vi "Image rotate and merge Main.vi"() -> ()   [LabVIEW 2016]
uses:
  <vilib>/vision/NI_Vision_Development_Module.lvlib
panel:
  out "最終角度":i32
  out "圖片數":i32
  in  "預設旋轉的步進角度":sgl=5.0
  out "提取範圍":T1(plugin-control)
  in  "預設 ROI":T2={"Rectangle"=[23, 116, 62, 596], "Contours"=[{"Type"=0, "ROI Type"=3, "Points"=[23, 116, 62, 596]}]}
  out "步進角度":sgl=3.8
  out "圖像中心位置":i32[](array[numeric])=[337, 356]
  out "圖像旋轉":T1(plugin-control)
  out "旋轉角度":sgl=22.8
  out "圖像合併":T1(plugin-control)
  in  "wait":u32=1000
  out "原始圖":T1(plugin-control)
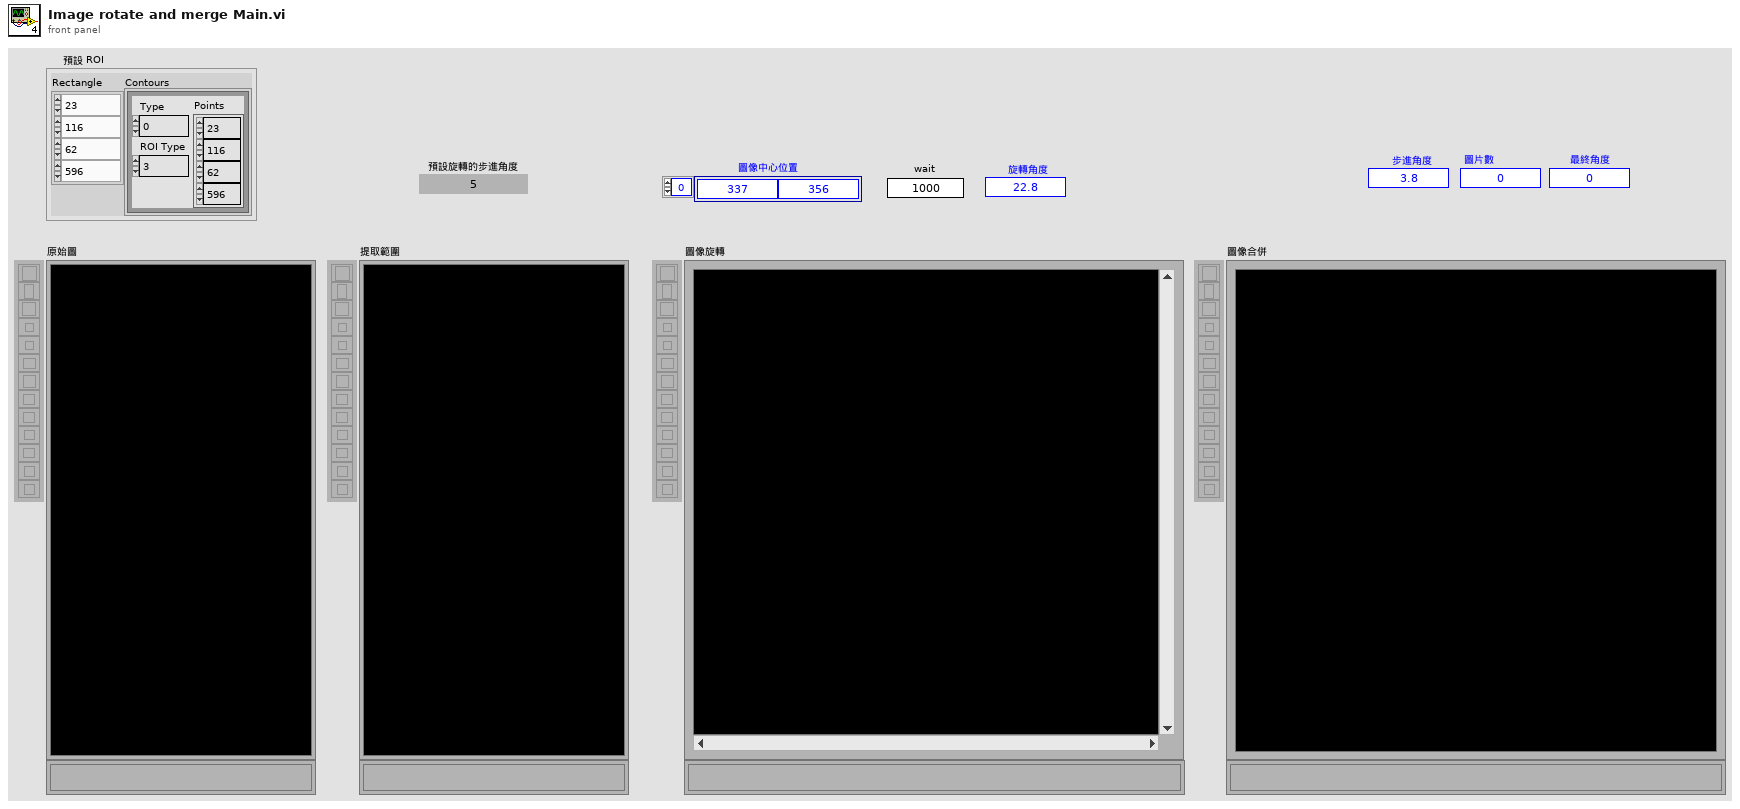
[diagram p1: front panel]
types:
  T1 = typedef "IMAQ Image.ctl" = refnum<image>
  T2 = cluster{"Rectangle":i32[], "Contours":cluster{"Type":u32, "ROI Type":u32, "Points":i32[]}[]}
  T3 = enum32{"Invalid", "Standard", "Closed", "Hidden", "Minimized", "Maximized"}
  T4 = cluster{"This VI":refnum<vi>, "path":path, "提取扇形矩形輪廓":i32[], "Roi 參數":cluster{"Left":i32, "Top":i32, "Right":i32, "Bottom":i32, "旋轉角度":sgl}, "中心點":cluster{"X":i32, "Y":i32}, "預設圖框":u8[][], "步進角度":sgl}
  T5 = cluster{"Global Rectangle":i32[], "Contours":cluster{"Contour Type":u32, "ROI Type":u32, "Points":i32[]}[]}
  T6 = typedef "IMAQ Rectangle" = cluster{"Left":i32, "Top":i32, "Right":i32, "Bottom":i32, "Rotation":dbl}
  T7 = typedef "Image Type" = u32
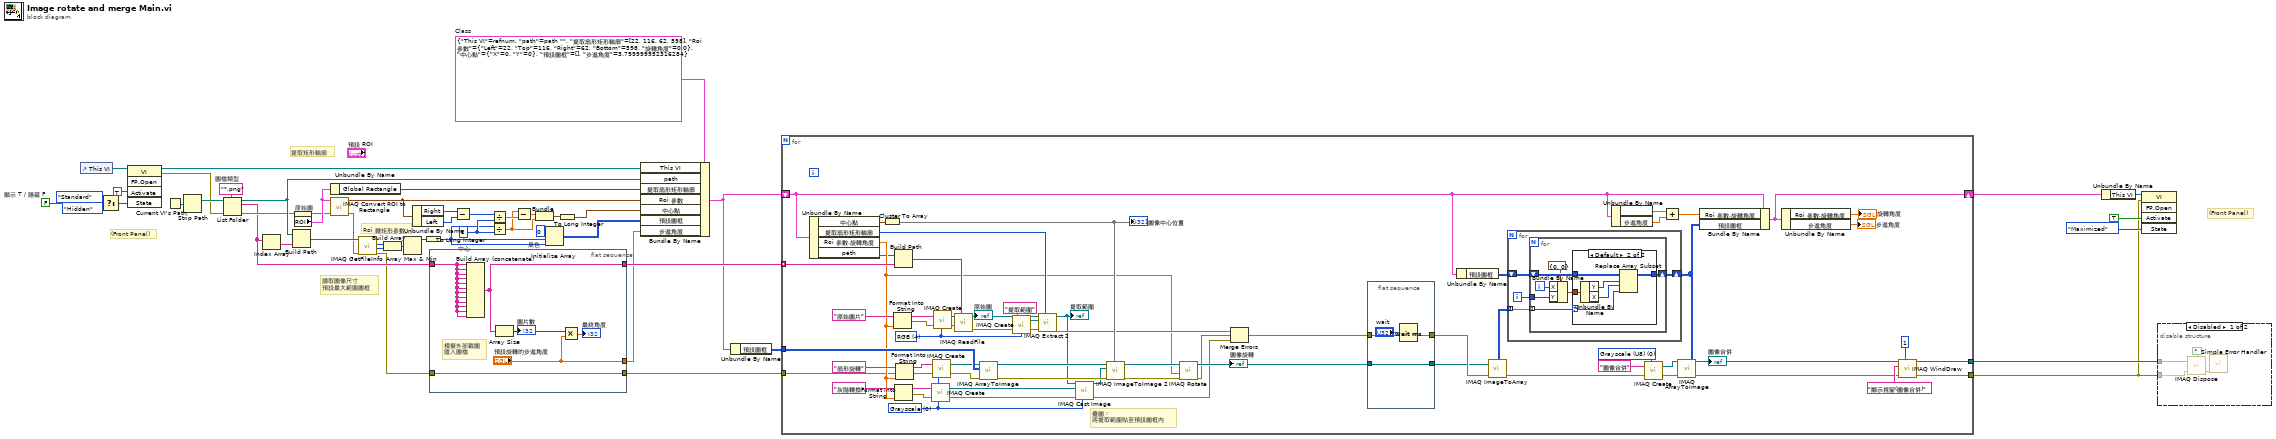
[diagram p0: block diagram]
diagram:
  w8 = FALSE  # 顯示 T / 隱藏 F
  w36 = 2  # 中心
  w42 = u8 0  # 黑色
  w28 = T4 {"This VI"=refnum, "path"=path "", "提取扇形矩形輪廓"=[22, 116, 62, 598], "Roi 參數"={"Left"=22, "Top"=116, "Right"=62, "Bottom"=598, "旋轉角度"=0.0}, "中心點"={"X"=0, "Y"=0}, "預設圖框"=[], "步進角度"=3.8}  # Class
  w48 = "*.png"  # 圖檔類型
  # "(Front Panel)"
  # "Roi 轉矩形參數"
  # "讀取圖像尺寸\n預設最大範圍圖框"
  # "(Front Panel)"
  # "提取矩形輪廓"
  n1 = control-ref of="This VI"() -> (w34:refnum<vi>)
  n2 = Select(t=T3."Standard" ("State"), s=w8, f=T3."Hidden" ("State")) -> (s? t:f=w5:T3)
  n3 = invoke class="VI" method="FP.Open"(reference=w34, "Activate"=TRUE ("Activate?"), "State"=w5) -> (reference out=w27:refnum<vi>, error out=w25:errorcluster)  [unwired: 2 in, 3 out]
  n4 = Current VI's Path() -> (path=w50:path)
  n5 = Strip Path(path=w50) -> (stripped path=w49:path)  [unwired: 1 out]
  n6 = List Folder(path=w49, pattern=w48, error in=w25) -> (path out=w26:path, filenames=w15:string[], error out=w23:errorcluster)  [unwired: 1 in, 1 out]
  n7 = Index Array(array=w15) -> (element=w47:string)  [unwired: 1 in]
  n8 = Build Path(base path=w26, name or relative path=w47) -> (appended path=w46:path)
  n9 = property on="原始圖" class="ImageControl"(error in=w23) -> (error out=w22:errorcluster, "ROI"=w24:T5)  [unwired: 1 in, 1 out]
  n10 = Unbundle By Name(w24) -> ("Global Rectangle"=w21:i32[])
  n11 = call "IMAQ Convert ROI to Rectangle"("error in (no error)"=w22, "ROI Descriptor"=w24) -> ("error out"=w4:errorcluster, "Rectangle"=w20:T6)  [unwired: 7 in]
  n12 = call "IMAQ GetFileInfo"("error in (no error)"=w4, "File Path"=w46) -> ("error out"=w3:errorcluster, "Y Resolution"=w43:i32, "X Resolution"=w45:i32)  [unwired: 3 in, 4 out]
  n13 = Build Array(w45, w43) -> (w44:i32[])
  n14 = Array Max & Min(array=w44) -> (max value=w41:i32)  [unwired: 3 out]
  n15 = Unbundle By Name(w20) -> ("Right"=w40:i32, "Left"=w39:i32)
  n16 = To Long Integer(number=w41) -> (32bit integer=w35:i32)
  n17 = flat-sequence {
    tunnel: w15 -> [w55]
    tunnel: [w53] -> w14
    tunnel: [w56] -> w13
    tunnel: w3 -> [w56]
    tunnel: ["預設旋轉的步進角度"] -> w9
    frame #0 {
      # "模擬外部截圖\n匯入圖檔"
      n18 = Build Array (concatenate)(w55, w55, w55, w55, w55, w55, w55, w55, w55, w55, w55, w55) -> (w53:string[])
      n19 = Array Size(array=w53) -> (size(s)=w54:i32)
      "圖片數" <- w54
      n20 = Multiply(x=w54, y="預設旋轉的步進角度") -> (x*y=→"最終角度":sgl)
    }
  }
  n21 = Subtract(x=w40, y=w39) -> (x-y=w38:i32)
  n22 = Divide(x=w38, y=w36) -> (x/y=w37:dbl)
  n23 = Divide(x=w35, y=w36) -> (x/y=w18:dbl)
  n24 = Subtract(x=w18, y=w37) -> (x-y=w19:dbl)
  n25 = Bundle(w19, w18) -> (w17:cluster{dbl, dbl})  [unwired: 1 in]
  n26 = Initialize Array(w42, w35, w35) -> (w11:u8[][])
  n27 = To Long Integer(number=w17) -> (32bit integer=w16:cluster{i32, i32})
  n28 = Bundle By Name(cluster=w28, "This VI"=w27, "path"=w26, "提取扇形矩形輪廓"=w21, "Roi 參數"=w20, "中心點"=w16, "預設圖框"=w11, "步進角度"=w9) -> (w12:T4)
  n29 = Unbundle By Name(w12) -> ("預設圖框"=w10:u8[][])
  n30 = for {
    tunnel: w14 -> [w115] mode=indexing
    tunnel: [w58] -> w1
    shift-right: [w70] -> w30
    shift-left: w12 -> [w93]
    tunnel: w10 -> [w92]
    tunnel: [w59] -> w2
    tunnel: w13 -> [w81]
    w110 = T7 0 items=["Grayscale (U8)", "Grayscale (I16)", "Grayscale (SGL)", "Complex (CSG)", "RGB (U32)", "HSL (U32)", "RGB (U64)", "Grayscale (U16)"] ("Image Type")
    w97 = T7 0 items=["Grayscale", "Grayscale (I16)", "Grayscale (SGL)", "Complex (CSG)", "RGB (U32)", "HSL (U32)", "RGB (U64)", "Grayscale (U16)"] ("Image Type")
    w71 = T7 4 items=["Grayscale (U8)", "Grayscale (I16)", "Grayscale (SGL)", "Complex (CSG)", "RGB", "HSL (U32)", "RGB (U64)", "Grayscale (U16)"] ("Image Type")
    # "疊圖 :\n將提取範圍貼至預設圖框內"
    n31 = Unbundle By Name(w93) -> ("中心點"=w85:cluster{"X":i32, "Y":i32}, "提取扇形矩形輪廓"=w84:i32[], "Roi 參數.旋轉角度"=w83:sgl, "path"=w82:path)
    n32 = Cluster To Array(cluster=w85) -> (array=w87:i32[])
    "圖像中心位置" <- w87
    n33 = Format Into String(initial string="原始圖片" ("Image Name"), w83) -> (resulting string=w120:string, error out=w119:errorcluster)  [unwired: 2 in]
    n34 = Format Into String(initial string="灰階轉換" ("Image Name"), w83) -> (resulting string=w117:string, error out=w116:errorcluster)  [unwired: 2 in]
    n35 = Build Path(base path=w82, name or relative path=w115) -> (appended path=w114:path)
    n36 = Format Into String(initial string="扇形旋轉" ("Image Name"), error in=w81, w83) -> (resulting string=w101:string, error out=w100:errorcluster)  [unwired: 1 in]
    n37 = call "IMAQ Create"("Image Name"=w117, "Image Type"=w97, "error in (no error)"=w116) -> ("New Image"=w111:T1, "error out"=w89:errorcluster)  [unwired: 1 in, 1 out]
    n38 = call "IMAQ Create"("Image Name"=w101, "Image Type"=w97, "error in (no error)"=w100) -> ("New Image"=w74:T1, "error out"=w103:errorcluster)  [unwired: 1 in, 1 out]
    n39 = call "IMAQ Create"("Image Name"=w120, "Image Type"=w71, "error in (no error)"=w119) -> ("New Image"=w113:T1, "error out"=w112:errorcluster)  [unwired: 2 in]
    n40 = call "IMAQ ReadFile"("File Path"=w114, "error in (no error)"=w112, "Image"=w113) -> ("error out"=w67:errorcluster, "Image Out"=w75:T1)  [unwired: 4 in, 3 out]
    "原始圖" <- w75
    n41 = call "IMAQ ArrayToImage"("error in (no error)"=w103, "Image Pixels (U8)"=w92, "Image"=w74) -> ("error out"=w98:errorcluster, "Image Out"=w99:T1)  [unwired: 7 in]
    n42 = call "IMAQ Create"("Image Name"="提取範圍", "Image Type"=w71, "error in (no error)"=w67) -> ("New Image"=w72:T1, "error out"=w66:errorcluster)  [unwired: 2 in]
    n43 = call "IMAQ Extract 2"("Optional Rectangle"=w84, "error in (no error)"=w66, "Image Dst"=w72, "Image Src"=w75) -> ("error out"=w86:errorcluster, "Image Dst Out"=w65:T1)  [unwired: 6 in]
    "提取範圍" <- w65
    n44 = call "IMAQ Cast Image"("Image Type"=w97, "error in (no error)"=w89, "Image Dst"=w111, "Image Src"=w65) -> ("error out"=w63:errorcluster, "Image Dst Out"=w73:T1)  [unwired: 6 in]
    n45 = call "IMAQ ImageToImage 2"("Offset Left/Top"=w87, "error in (no error)"=w98, "Image Src (Small)"=w73, "Image Src (Large)"=w99) -> ("error out"=w104:errorcluster, "Image Dst Out"=w105:T1)  [unwired: 6 in]
    n46 = call "IMAQ Rotate"("error in (no error)"=w104, "Angle (degrees)"=w83, "Image Src"=w105) -> ("error out"=w64:errorcluster, "Image Dst Out"=w78:T1)  [unwired: 7 in]
    "圖像旋轉" <- w78
    n47 = Merge Errors(w86, w64, w63) -> (w79:errorcluster)
    n48 = flat-sequence {
      tunnel: [w123] -> w80
      tunnel: w79 -> [w123]
      tunnel: [w122] -> w77
      tunnel: w78 -> [w122]
      frame #0 {
        n49 = Wait (ms)(milliseconds to wait="wait") -> ()  [unwired: 1 out]
      }
    }
    n50 = Unbundle By Name(w93) -> ("預設圖框"=w96:u8[][])
    n51 = call "IMAQ ImageToArray"("error in (no error)"=w80, "Image"=w77) -> ("error out"=w107:errorcluster, "Image Pixels (U8)"=w106:u8[][])  [unwired: 2 in, 3 out]
    n52 = for {
      tunnel: w106 -> [w126] mode=indexing
      shift-right: [w127] -> w95
      shift-left: w96 -> [w128]
      i -> [w125]
      n53 = for {
        tunnel: w126 -> [w131] mode=indexing
        tunnel: w125 -> [w130]
        shift-right: [w134] -> w127
        shift-left: w128 -> [w135]
        i -> [w132]
        n54 = Bundle By Name(cluster=cluster{"X":i32, "Y":i32} {"X"=0, "Y"=0} ("像素座標"), "X"=w132, "Y"=w130) -> (w129:cluster{"X":i32, "Y":i32})
        n55 = case shown="Default" w131 {
          selector: w131 -> [_ w138]
          tunnel: w135 -> [w136 w142]
          tunnel: [w136 w141] -> w134
          tunnel: w129 -> [_ w140]
          frame 0..50 {
          }
          frame Default {
            n56 = Unbundle By Name(w140) -> ("Y"=w137:i32, "X"=w139:i32)
            n57 = Replace Array Subset(array=w142, new element=w138, index (row)=w137, index (col)=w139) -> (w141:u8[][])
          }
        }
      }
    }
    n58 = Unbundle By Name(w93) -> ("Roi 參數.旋轉角度"=w94:sgl, "步進角度"=w91:sgl)
    n59 = call "IMAQ Create"("Image Name"="圖像合併", "Image Type"=w110, "error in (no error)"=w107) -> ("New Image"=w108:T1, "error out"=w88:errorcluster)  [unwired: 1 in, 1 out]
    n60 = Add(x=w94, y=w91) -> (x+y=w90:sgl)
    n61 = call "IMAQ ArrayToImage"("error in (no error)"=w88, "Image Pixels (U8)"=w95, "Image"=w108) -> ("error out"=w60:errorcluster, "Image Out"=w61:T1)  [unwired: 7 in]
    "圖像合併" <- w61
    n62 = Bundle By Name(cluster=w93, "Roi 參數.旋轉角度"=w90, "預設圖框"=w95) -> (w70:T4)
    n63 = Unbundle By Name(w70) -> ("Roi 參數.旋轉角度"=→"旋轉角度":sgl, "步進角度"=→"步進角度":sgl)
    n64 = call "IMAQ WindDraw"("Window Number (0...15)"=1, "error in (no error)"=w60, "Title"="顯示視窗(圖像合併)", "Image"=w61) -> ("error out"=w58:errorcluster, "Image Out (duplicate)"=w59:T1)  [unwired: 6 in]
  }
  n65 = Unbundle By Name(w30) -> ("This VI"=w29:refnum<vi>)
  n66 = invoke class="VI" method="FP.Open"(reference=w29, error in=w1, "Activate"=TRUE ("Activate?"), "State"=T3."Maximized") -> ()  [unwired: 1 in, 5 out]
  n67 = disable-structure shown="Disabled" {
    disable-tunnel: w2 -> [w145 _]
    disable-tunnel: w1 -> [w143 _]
    frame Disabled {
      n68 = call "IMAQ Dispose"("All Images? (No)"=FALSE, "Image"=w145, "error in (no error)"=w143) -> ("error out"=w144:errorcluster)  [unwired: 3 in]
      n69 = call <vilib>:"Simple Error Handler.vi"("error in (no error)"=w144) -> ()  [unwired: 4 in, 5 out]
    }
    frame Enabled {
    }
  }
